vi "CoboltLaser_TempGet.vi"(8 "ErrorIn":errorcluster, 10 "CheckResponse":bool=TRUE, 11 "ComPort":refnum<visa-resource-name>) -> (0 "ErrorOut":errorcluster, 1 "Température":dbl, 2 "Response":string, 3 "ComPortOut":refnum<visa-resource-name>, 4 "ResponseOK":bool)   [LabVIEW 2019]
doc: "Use this template to build a VI to use as a subVI."
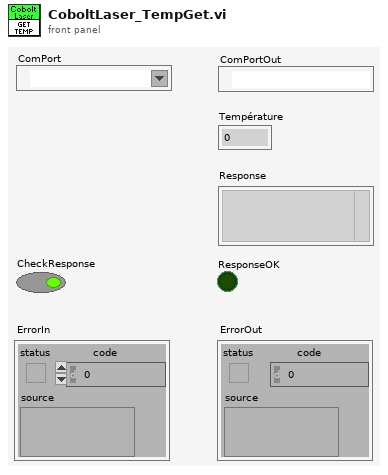
[diagram p1: front panel]
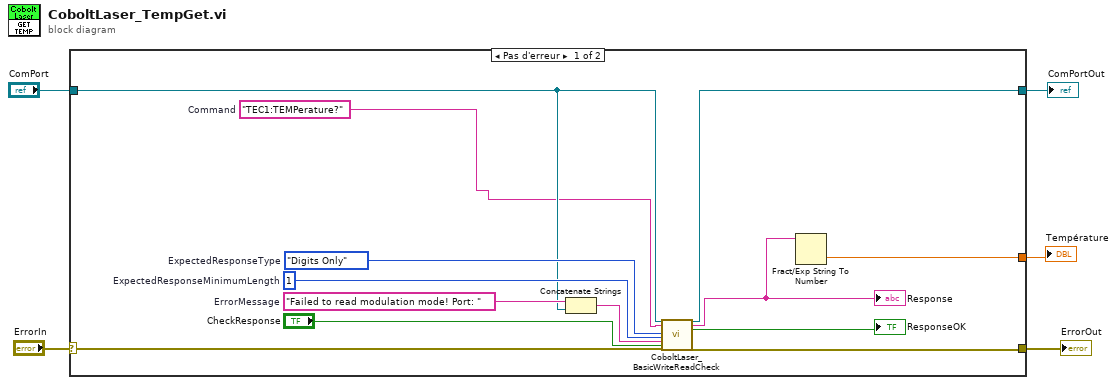
[diagram p0: block diagram]
diagram:
  n1 = case shown="Pas d'erreur" "ErrorIn" {
    selector: "ErrorIn" -> [w18 w20]
    tunnel: [w17 w20] -> w4
    tunnel: "ComPort" -> [w10 w19]
    tunnel: [w9 w19] -> w2
    tunnel: [w6 _] -> w1
    frame No Error {
      w7 = "TEC1:TEMPerature?"  # Command
      w15 = 1  # ExpectedResponseMinimumLength
      w16 = enum16{"Any", "Digits Only", "Non-Digits Only"}."Digits Only"  # ExpectedResponseType
      w12 = "Failed to read modulation mode! Port: "  # ErrorMessage
      n2 = Concatenate Strings(w12, w10) -> (w11:string)
      n3 = call <userlib>:"CoboltLaser_BasicWriteReadCheck.vi"("ComPort"=w10, "Command"=w7, "ExpectedResponseType"=w16, "ExpectedResponseMinimumLength"=w15, "ErrorMessage"=w11, "GenerateError"="CheckResponse", "error in (no error)"=w18) -> ("ComPortOut"=w9:refnum<visa-resource-name>, "Response"=w8:string, "ResponseOK"=→"ResponseOK":bool, "error out"=w17:errorcluster)  [unwired: 17 in]
      "Response" <- w8
      n4 = Fract/Exp String To Number(string=w8) -> (number=w6:dbl)  [unwired: 3 in, 1 out]
    }
    frame Error {
    }
  }
  "ErrorOut" <- w4
  "ComPortOut" <- w2
  "Température" <- w1
